vi "Example_OE2031&OE2041 Trig in.vi"() -> ()   [LabVIEW 2011]
panel:
  out "data_buffer":dbl[][](array[numeric])
  out "loss count":i32=-1
  out "cnt":u16
  in  "Ref_Source":u8(ring) items=["External", "Internal"]
  in  "Interval Count":u32=1 min=1 max=100000
  in  "选项卡控件":enum32{"选项卡 "}(tab)
  in  "Sweep Mode":u16(ring) items=["Linear", "Log"]
  in  "Start Frequency(Hz)":dbl=1000.0 min=1e-05 max=60000000.0 format="%#.3f"
  in  "Stop Frequency(Hz)":dbl=5000.0 min=1e-05 max=60000000.0 format="%#.3f"
  in  "Linear Step Frequency(Hz)":dbl=1000.0 min=1e-05 max=60000000.0 format="%#.3f"
  in  "Log Step Percent(%)":dbl=10.0 min=-100.0 max=100.0 format="%#.2f"
  in  "Step Time(ms)":i32=1000 min=50 max=100000
  in  "Sweep Run Mode":u16(ring) items=["Stop", "Singal", "Loop"]
  out "Group":u32
  in  "Sweep":u16(ring) items=["OFF", "ON"]
  in  "function":T1(ring)
  in  "Parameter Index":u16(ring) items=["X", "Y", "R", "θ", "Frequency", "XD1", "YD1", "RD1", "θD1", "XD2", "YD2", "RD2", "θD2", "XD3", "YD3", "RD3", "θD3", "X_Noise", "Y_Noise", "AUXADC1", "AUXADC2", "AUXADC3", "AUXADC4"]
  out "Wave":dbl(graph)
  in  "IP Address":string="192.168.1.10"
  in  "Timeout":u32=100
  in  "Port":u32=10001
  in  "Connect":bool
  in  "Trig Mode":u8(ring) items=["Internal", "Ext_Rissing_Edge", "Ext_Falling_Edge", "Ext_High_Level", "Ext_Low_Level"]
  out "Error out":errorcluster caption="error out"
  in  "Remote Mode":u16(ring) items=["USB"=0, "Ethernet"=3]
  in  "VISA resource name":refnum<visa-resource-name>
  # "Tel          :   +86-020-84133345\nWebsite  :   www.ssi-instrument.com\nE-mail     :   support@si-instrument.com"
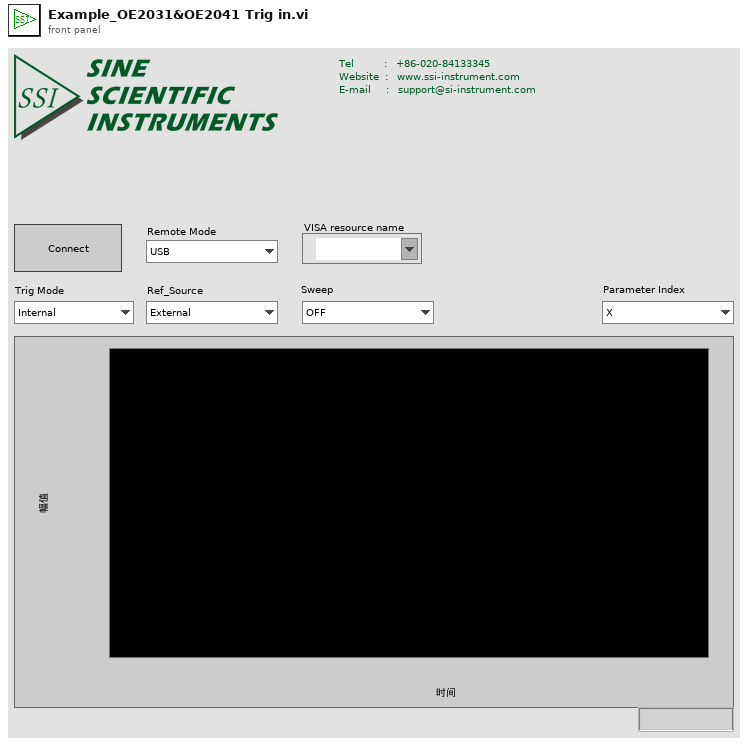
[diagram p1: front panel]
types:
  T1 = enum16{"initial", "Trig In Type", "Sample", "Ext_Sweep_Trig In", "Int_Sweep_Trig In"}
  T2 = enum8{"Enabled", "Disabled", "Disabled and Grayed Out"}
  T3 = cluster{"Port":u32, "Timeout":u32, "IP Address":string}
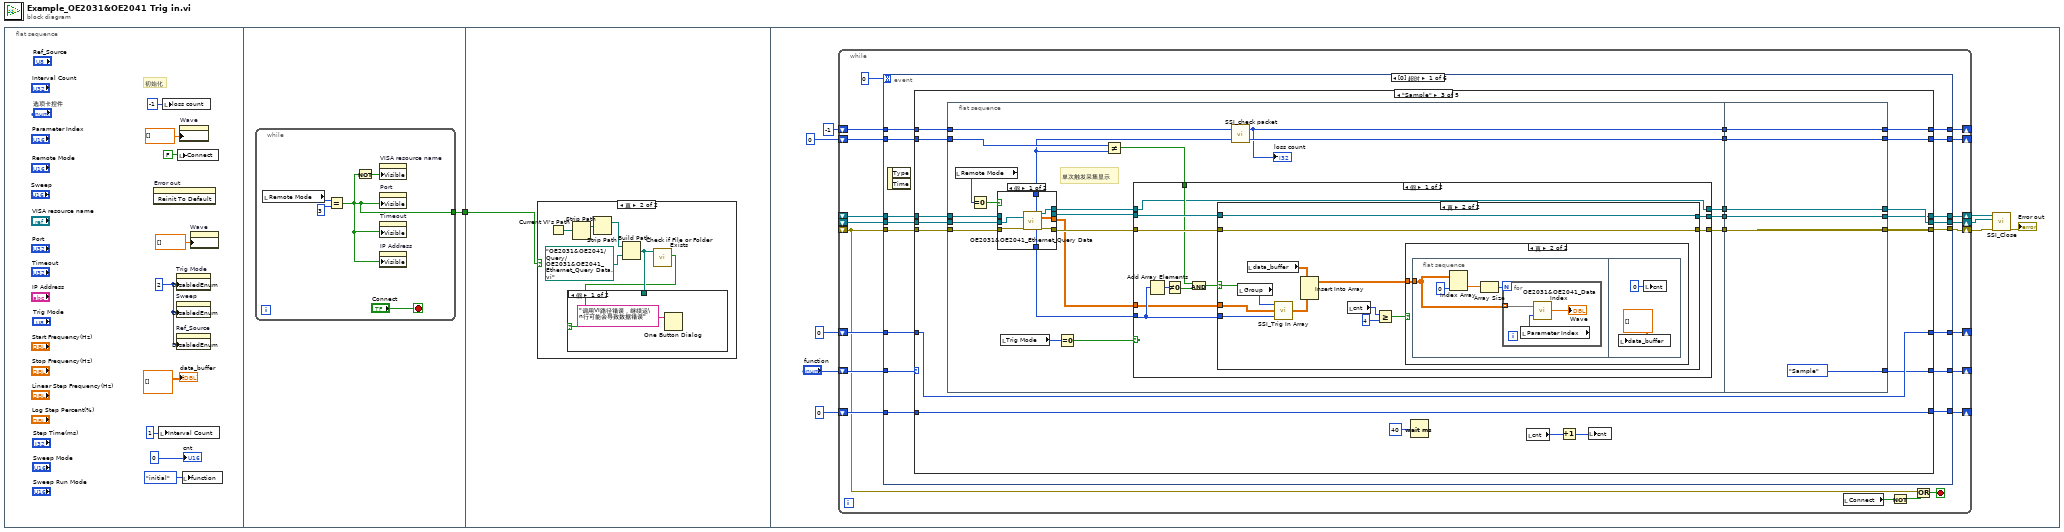
[diagram p0: block diagram]
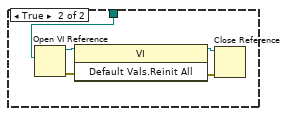
[diagram p3: hidden frame]
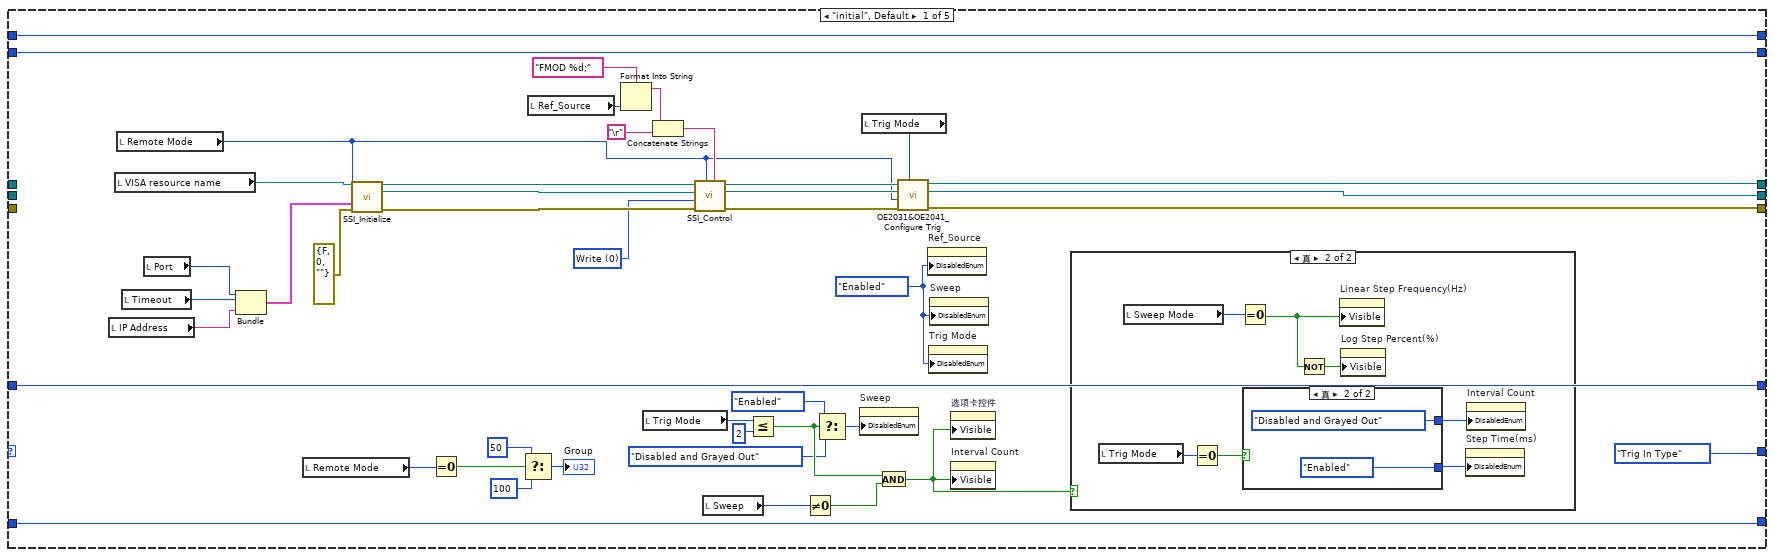
[diagram p4: hidden frame]
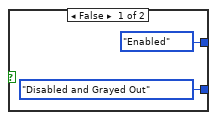
[diagram p6: hidden frame]
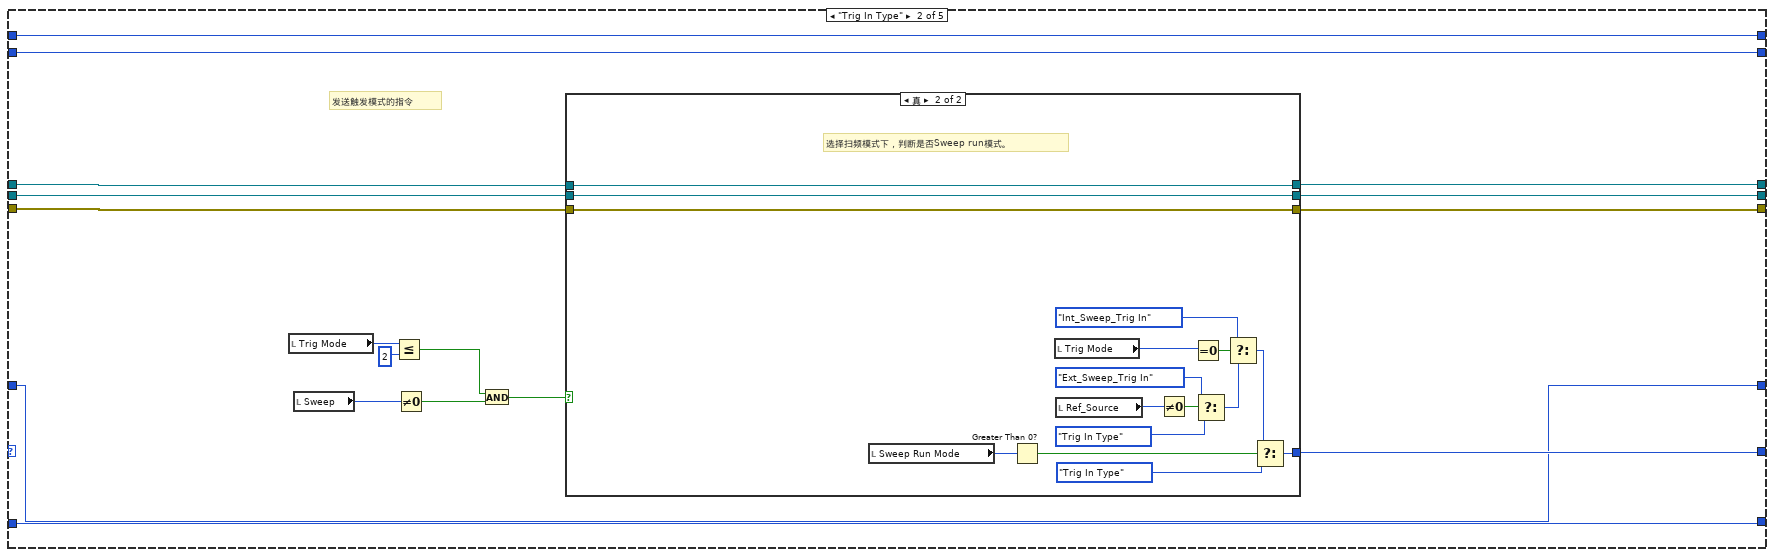
[diagram p7: hidden frame]
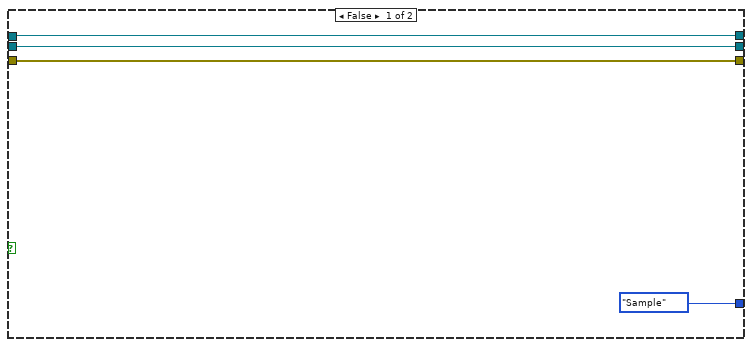
[diagram p8: hidden frame]
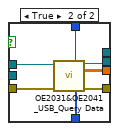
[diagram p9: hidden frame]
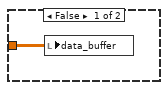
[diagram p11: hidden frame]
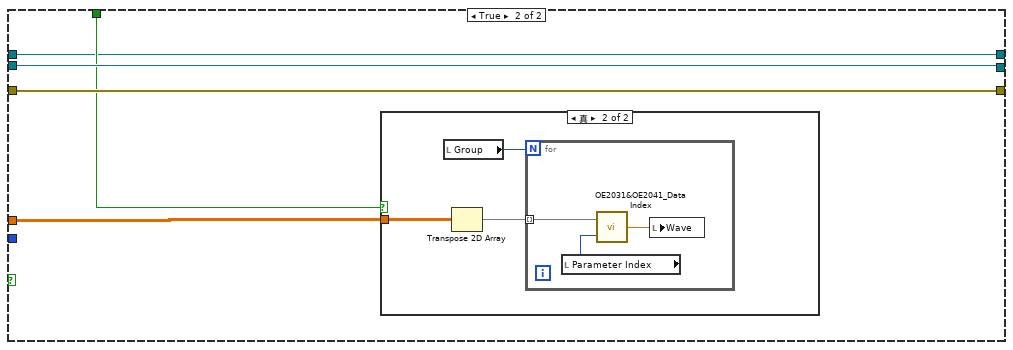
[diagram p12: hidden frame]
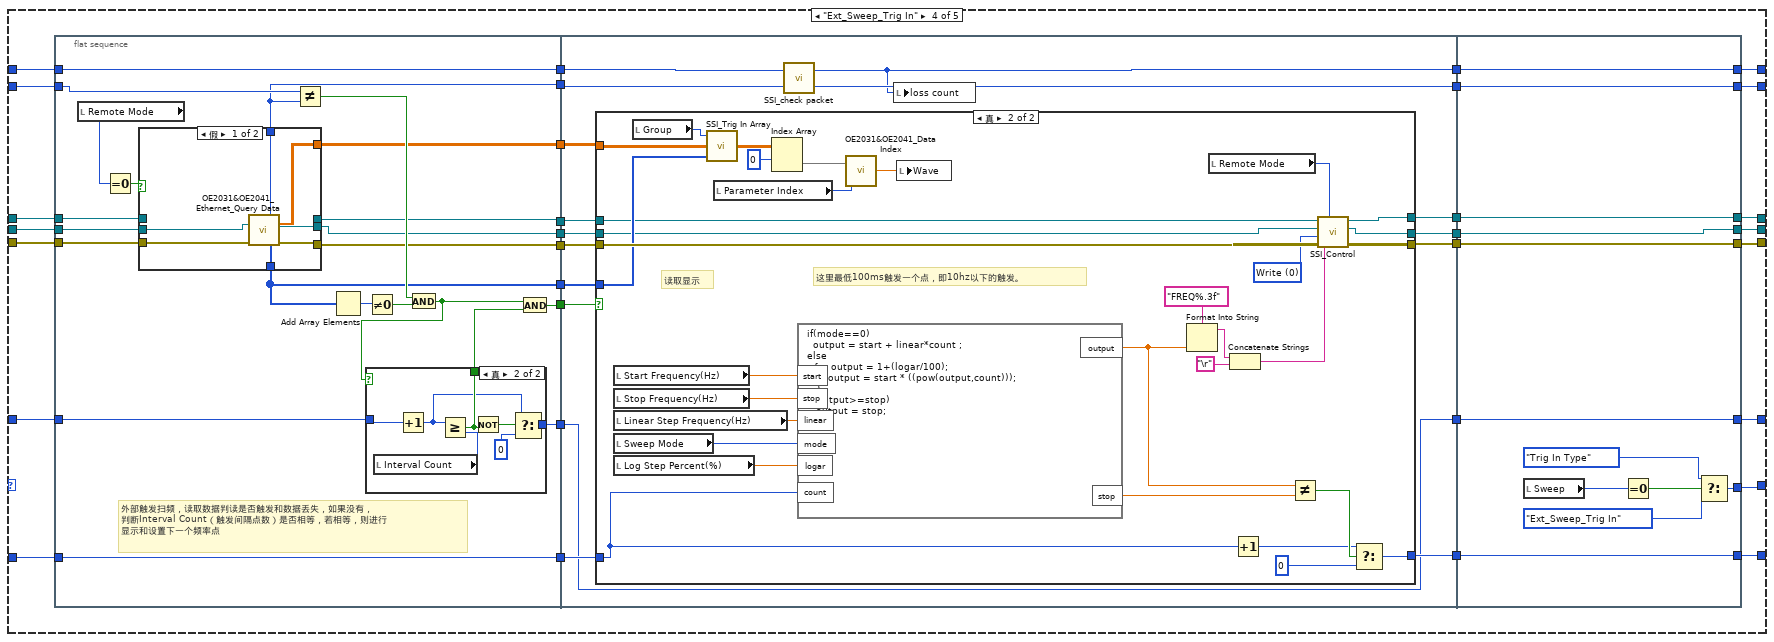
[diagram p14: hidden frame]
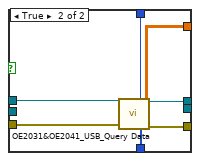
[diagram p15: hidden frame]
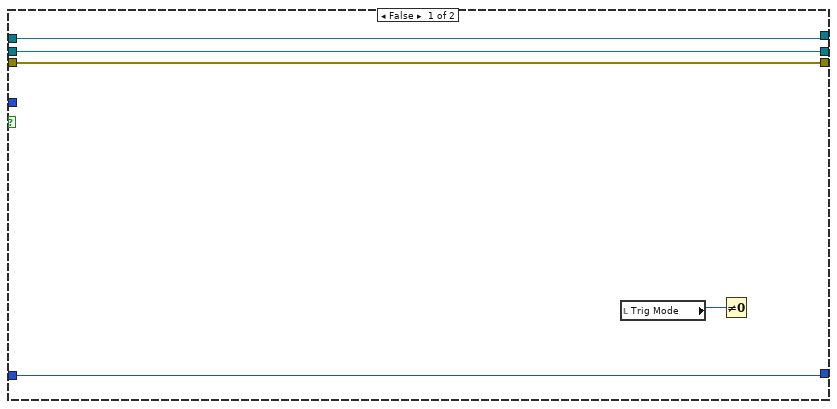
[diagram p17: hidden frame]
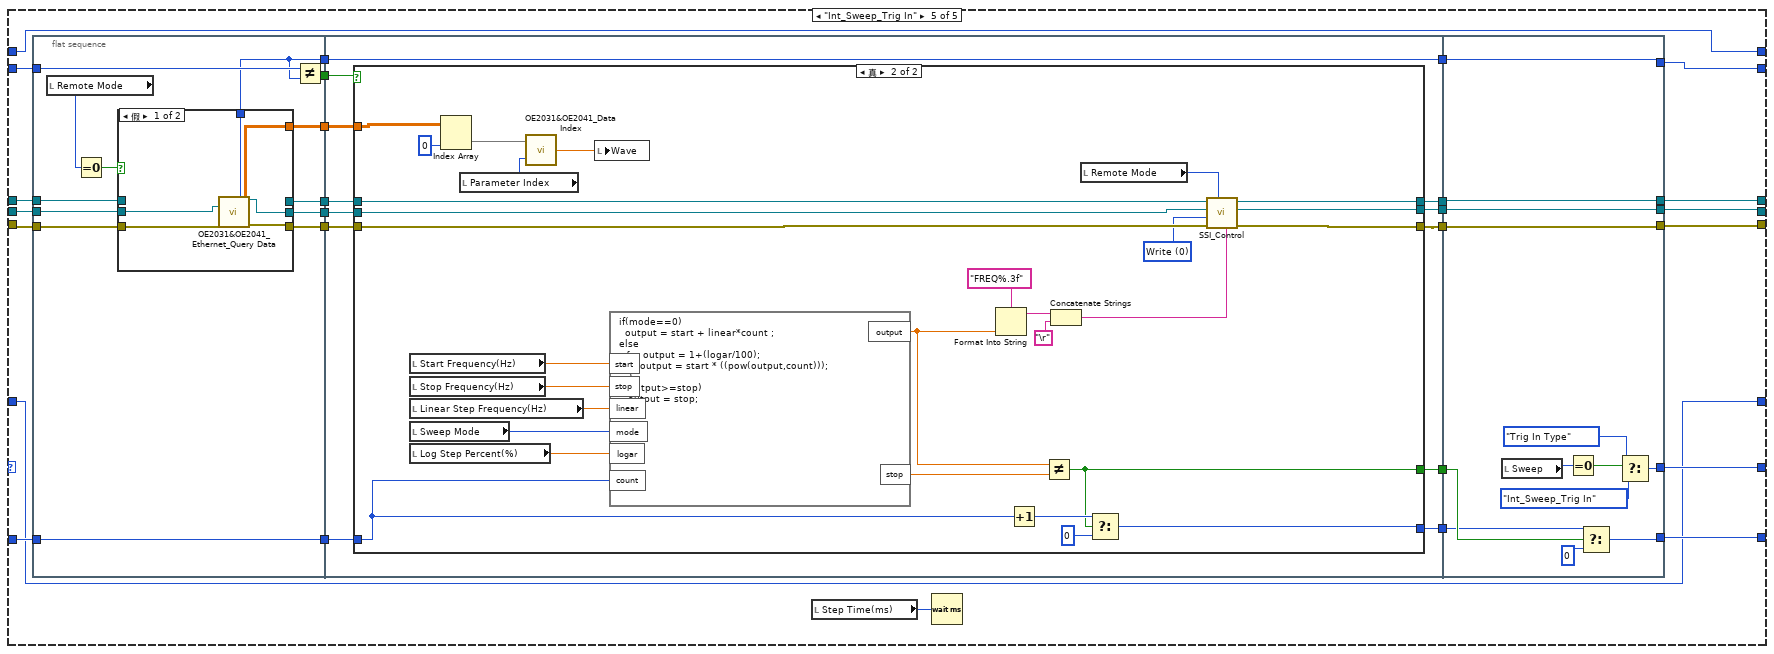
[diagram p18: hidden frame]
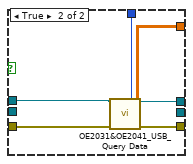
[diagram p19: hidden frame]
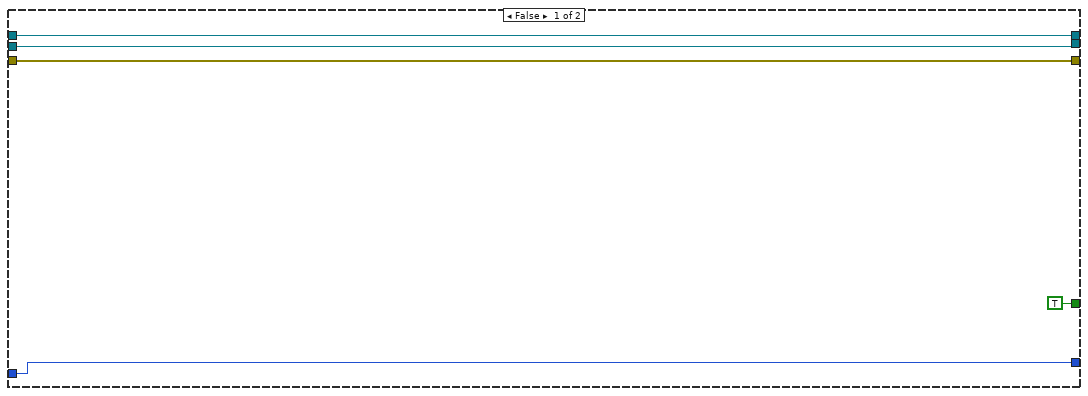
[diagram p20: hidden frame]
diagram:
  n1 = flat-sequence {
    tunnel: [w11] -> w1
    tunnel: w1 -> [w17]
    frame #0 {
      w3 = 2
      # "初始化"
      n2 = invoke on="Error out" class="Clust (严格)" method="Reinit To Default"() -> ()  [unwired: 3 in, 3 out]
      n3 = local write "Interval Count"(u32 1 ("Interval Count")) -> ()
      n4 = local write "loss count"(-1 ("loss count")) -> ()
      n5 = property on="Trig Mode" class="Ring (严格)"("DisabledEnum"=w3) -> ()  [unwired: 2 in, 2 out]
      n6 = property on="Sweep" class="Ring (严格)"("DisabledEnum"=w3) -> ()  [unwired: 2 in, 2 out]
      n7 = property on="Ref_Source" class="Ring (严格)"("DisabledEnum"=w3) -> ()  [unwired: 2 in, 2 out]
      n8 = local write "Connect"(FALSE ("Connect")) -> ()
      n9 = property on="Wave" class="WFChart (严格)"("History Data"=dbl[] [] ("历史数据")) -> ()  [unwired: 2 in, 2 out]
      n10 = local write "function"(T1."initial" ("function")) -> ()
      n11 = property on="Wave" class="WFChart (严格)"("History Data"=dbl[] [] ("历史数据")) -> ()  [unwired: 2 in, 2 out]
      "data_buffer" <- dbl[][] []
      "cnt" <- 0
    }
    frame #1 {
      n12 = while {
        tunnel: [w12] -> w11
        stop <- "Connect" stop-if-true
        n13 = local read "Remote Mode"() -> (w15:u16)
        n14 = Equal?(x=w15, y=u16 3) -> (x = y?=w12:bool)
        n15 = Not(x=w12) -> (.not. x?=w13:bool)
        n16 = property on="VISA resource name" class="VISAName"("Visible"=w13) -> ()  [unwired: 2 in, 2 out]
        n17 = property on="Port" class="DigNum (严格)"("Visible"=w12) -> ()  [unwired: 2 in, 2 out]
        n18 = property on="Timeout" class="DigNum (严格)"("Visible"=w12) -> ()  [unwired: 2 in, 2 out]
        n19 = property on="IP Address" class="Str"("Visible"=w12) -> ()  [unwired: 2 in, 2 out]
      }
    }
    frame #2 {
      n20 = case shown="真" w17 {
        frame False {
        }
        frame True {
          n21 = Current VI's Path() -> (path=w19:path)
          n22 = Strip Path(path=w19) -> (stripped path=w18:path)  [unwired: 1 out]
          n23 = Strip Path(path=w18) -> (stripped path=w20:path)  [unwired: 1 out]
          n24 = Build Path(base path=w20, name or relative path=path "OE2031&OE2041/Query/OE2031&OE2041_Ethernet_Query Data.vi") -> (appended path=w23:path)
          n25 = call <vilib>:"Check if File or Folder Exists.vi"("path"=w23) -> ("file or folder exists?"=w21:bool)  [unwired: 8 in, 2 out]
          n26 = case shown="假" w21 {
            tunnel: w23 -> [_ w29]
            frame False {
              n27 = One Button Dialog(message="调用VI路径错误，继续运\n行可能会导致数据错误" ("消息")) -> ()  [unwired: 1 in, 1 out]
            }
            frame True {
              n28 = Open VI Reference(vi path=w29) -> (vi reference=w26:refnum<vi>, error out=w25:errorcluster)  [unwired: 5 in]
              n29 = invoke class="VI" method="Default Vals.Reinit All"(reference=w26, error in=w25) -> (reference out=w28:refnum<vi>, error out=w27:errorcluster)  [unwired: 1 in, 1 out]
              n30 = Close Reference(reference=w28, error in (no error)=w27) -> ()  [unwired: 1 out]
            }
          }
        }
      }
    }
    frame #3 {
      n31 = while {
        shift-right: [w53] -> _
        shift-left: "function" -> [w54]
        shift-right: [w51] -> _
        shift-left: 0 ("f") -> [w52]
        shift-right: [w48] -> _
        shift-left: 0 -> [w49]
        shift-right: [w45] -> _
        shift-left: 0 -> [w46]
        shift-right: [w42] -> w32
        shift-left: _ -> [w56]
        shift-right: [w55] -> w37
        shift-left: _ -> [w44]
        shift-right: [w43] -> w33
        shift-left: _ -> [w41]
        shift-right: [w39] -> _
        shift-left: -1 ("loss count") -> [w40]
        stop <- w57 stop-if-true
        n32 = event shown="[0] 超时" {
          selector: _ -> [_ _ _ _ _ _]
          dyn-events: _ -> [_ _ _ _ _ _]
          timeout: 0 -> [_ _ _ _ _ _]
          tunnel: w56 -> [w74 w529 w541 w560 w586 w605]
          tunnel: [w73 w529 w541 w555 w585 w605] -> w42
          tunnel: [w72 w527 w540 w557 w588 w606] -> w55
          tunnel: w44 -> [w71 w527 w540 w562 w589 w606]
          tunnel: w54 -> [w70 _ _ _ w592 _]
          tunnel: [w69 T1."Trig In Type" ("function") T1."Trig In Type" ("function") T1."Trig In Type" ("function") w592 T1."Trig In Type" ("function")] -> w53
          tunnel: w52 -> [w68 w533 w543 w567 w593 w601]
          tunnel: [w67 w533 w543 w567 w593 w601] -> w51
          tunnel: w49 -> [w66 w531 w538 w565 w590 w603]
          tunnel: [w65 w531 w538 w565 w590 w603] -> w48
          tunnel: w46 -> [w64 w524 w537 w566 w591 w600]
          tunnel: [w63 w524 w537 w566 w591 w600] -> w45
          tunnel: [w62 w528 w535 w556 w584 w604] -> w43
          tunnel: w41 -> [w61 w528 w535 w561 w587 w604]
          tunnel: w40 -> [w60 w530 w534 w544 w579 w602]
          tunnel: [w59 w530 w534 w544 w579 w602] -> w39
          event Timeout {
            n33 = event-data() -> ()  [unwired: 1 in, 2 out]
            n34 = case shown="\"Sample\"" w70 {
              tunnel: w74 -> [_ w145 w185 w304 w424]
              tunnel: w71 -> [_ w143 w184 w303 w423]
              tunnel: [w96 w144 w168 w300 w437] -> w73
              tunnel: [w94 w142 w176 w301 w436] -> w72
              tunnel: [T1."Trig In Type" ("function") w141 w182 w289 w434] -> w69
              tunnel: w68 -> [w111 w140 w186 w302 w435]
              tunnel: [w111 w140 w186 w299 w433] -> w67
              tunnel: w66 -> [w109 w139 w181 w298 w439]
              tunnel: [w109 w139 w179 w297 w438] -> w65
              tunnel: w64 -> [w110 w138 w183 w284 w432]
              tunnel: [w110 w138 w183 w281 w432] -> w63
              tunnel: [w95 w130 w169 w277 w415] -> w62
              tunnel: w61 -> [_ w131 w171 w280 w419]
              tunnel: w60 -> [w76 w129 w174 w276 w414]
              tunnel: [w76 w129 w167 w273 w414] -> w59
              frame "initial", Default {
                w75 = T2."Enabled" ("禁用")
                w88 = u16 0 items=["Write", "Read"] ("Control")
                n35 = local read "IP Address"() -> (w91:string)
                n36 = local read "VISA resource name"() -> (w97:refnum<visa-resource-name>)
                n37 = local read "Remote Mode"() -> (w77:u16)
                n38 = local read "Timeout"() -> (w92:u32)
                n39 = local read "Port"() -> (w93:u32)
                n40 = Bundle("Port"=w93, "Timeout"=w92, "IP Address"=w91) -> (w90:T3)  [unwired: 1 in]
                n41 = local read "Remote Mode"() -> (w117:u16)
                n42 = call "SSI_Initialize.vi"("VISA resource name"=w97, "Remote Mode"=w77, "Ethernet"=w90, "error in (no error)"=errorcluster {"status"=FALSE, "code"=0, "source"=""}) -> ("VISA resource name out"=w101:refnum<visa-resource-name>, "connection ID(Ethernet)"=w102:refnum<k5>, "error out"=w98:errorcluster)  [unwired: 9 in]
                n43 = Equal To 0?(x=w117) -> (x = 0?=w113:bool)
                n44 = Select(t=50, s=w113, f=100) -> (s? t:f=→"Group":i32)
                n45 = local read "Ref_Source"() -> (w107:u8)
                n46 = Format Into String(format string="FMOD %d;" ("格式字符串"), w107) -> (resulting string=w108:string)  [unwired: 2 in, 1 out]
                n47 = local read "Trig Mode"() -> (w83:u8)
                n48 = Concatenate Strings(w108, "\r") -> (w87:string)
                n49 = call "SSI_Control.vi"("Write Buffer"=w87, "Remote Mode"=w77, "Error in (no error)"=w98, "Control"=w88, "Connection ID in"=w102, "VISA resource name"=w101) -> ("Error out"=w99:errorcluster, "Connection ID out"=w100:refnum<k5>, "VISA resource  out"=w103:refnum<visa-resource-name>)  [unwired: 2 in, 1 out]
                n50 = local read "Sweep"() -> (w84:u16)
                n51 = Less Or Equal?(x=w83, y=u8 2) -> (x <= y?=w85:bool)
                n52 = Not Equal To 0?(x=w84) -> (x != 0?=w86:bool)
                n53 = Select(t=T2."Enabled" ("禁用"), s=w85, f=T2."Disabled and Grayed Out") -> (s? t:f=w80:T2)
                n54 = property on="Sweep" class="Ring (严格)"("DisabledEnum"=w80) -> ()  [unwired: 2 in, 2 out]
                n55 = local read "Trig Mode"() -> (w104:u8)
                n56 = And(x=w85, y=w86) -> (x .and. y?=w78:bool)
                n57 = call "OE2031&OE2041_Configure Trig.vi"("Trig Mode"=w104, "Error in (no error)"=w99, "Remote Mode"=w77, "Connection ID in"=w100, "VISA resource name"=w103) -> ("Error out"=w94:errorcluster, "Connection ID out"=w95:refnum<k5>, "VISA resource  out"=w96:refnum<visa-resource-name>)  [unwired: 3 in, 1 out]
                n58 = property on="Ref_Source" class="Ring (严格)"("DisabledEnum"=w75) -> ()  [unwired: 2 in, 2 out]
                n59 = property on="Trig Mode" class="Ring (严格)"("DisabledEnum"=w75) -> ()  [unwired: 2 in, 2 out]
                n60 = property on="Sweep" class="Ring (严格)"("DisabledEnum"=w75) -> ()  [unwired: 2 in, 2 out]
                n61 = property on="选项卡控件" class="TabCtl (严格)"("Visible"=w78) -> ()  [unwired: 2 in, 2 out]
                n62 = property on="Interval Count" class="DigNum (严格)"("Visible"=w78) -> ()  [unwired: 2 in, 2 out]
                n63 = case shown="真" w78 {
                  frame False {
                  }
                  frame True {
                    n64 = local read "Trig Mode"() -> (w118:u8)
                    n65 = local read "Sweep Mode"() -> (w123:u16)
                    n66 = Equal To 0?(x=w118) -> (x = 0?=w119:bool)
                    n67 = Equal To 0?(x=w123) -> (x = 0?=w124:bool)
                    n68 = case shown="真" w119 {
                      tunnel: [T2."Disabled and Grayed Out" ("禁用") T2."Enabled" ("禁用")] -> w121
                      tunnel: [T2."Enabled" ("禁用") T2."Disabled and Grayed Out" ("禁用")] -> w120
                      frame False {
                      }
                      frame True {
                      }
                    }
                    n69 = Not(x=w124) -> (.not. x?=w122:bool)
                    n70 = property on="Linear Step Frequency(Hz)" class="DigNum (严格)"("Visible"=w124) -> ()  [unwired: 2 in, 2 out]
                    n71 = property on="Log Step Percent(%)" class="DigNum (严格)"("Visible"=w122) -> ()  [unwired: 2 in, 2 out]
                    n72 = property on="Step Time(ms)" class="DigNum (严格)"("DisabledEnum"=w121) -> ()  [unwired: 2 in, 2 out]
                    n73 = property on="Interval Count" class="DigNum (严格)"("DisabledEnum"=w120) -> ()  [unwired: 2 in, 2 out]
                  }
                }
              }
              frame "Trig In Type" {
                # "发送触发模式的指令"
                n74 = local read "Trig Mode"() -> (w135:u8)
                n75 = local read "Sweep"() -> (w134:u16)
                n76 = Less Or Equal?(x=w135, y=u8 2) -> (x <= y?=w133:bool)
                n77 = Not Equal To 0?(x=w134) -> (x != 0?=w132:bool)
                n78 = And(x=w133, y=w132) -> (x .and. y?=w137:bool)
                n79 = case shown="真" w137 {
                  tunnel: [w149 w161] -> w144
                  tunnel: [w148 w160] -> w142
                  tunnel: w143 -> [w148 w160]
                  tunnel: w145 -> [w149 w161]
                  tunnel: [T1."Sample" ("function") w164] -> w141
                  tunnel: w131 -> [w146 w150]
                  tunnel: [w146 w150] -> w130
                  frame False {
                  }
                  frame True {
                    # "选择扫频模式下，判断是否Sweep run模式。"
                    n80 = local read "Sweep Run Mode"() -> (w162:u16)
                    n81 = Greater Than 0?(x=w162) -> (x > 0?=w165:bool)
                    n82 = local read "Trig Mode"() -> (w155:u8)
                    n83 = local read "Ref_Source"() -> (w159:u8)
                    n84 = Not Equal To 0?(x=w159) -> (x != 0?=w158:bool)
                    n85 = Equal To 0?(x=w155) -> (x = 0?=w156:bool)
                    n86 = Select(t=T1."Ext_Sweep_Trig In" ("function"), s=w158, f=T1."Trig In Type" ("function")) -> (s? t:f=w157:T1)
                    n87 = Select(t=T1."Int_Sweep_Trig In" ("function"), s=w156, f=w157) -> (s? t:f=w163:T1)
                    n88 = Select(t=w163, s=w165, f=T1."Trig In Type" ("function")) -> (s? t:f=w164:T1)
                  }
                }
              }
              frame "Sample" {
                n89 = flat-sequence {
                  tunnel: w185 -> [w205]
                  tunnel: w184 -> [w204]
                  tunnel: w181 -> [w201]
                  tunnel: [w197] -> w180
                  tunnel: [w199] -> w178
                  tunnel: [w198] -> w177
                  tunnel: w174 -> [w196]
                  tunnel: w171 -> [w192]
                  tunnel: [w189] -> w170
                  tunnel: [w188] -> w166
                  tunnel: w180 -> [w268]
                  tunnel: w178 -> [w272]
                  tunnel: w177 -> [w271]
                  tunnel: [T1."Sample" ("function")] -> w182
                  tunnel: [w268] -> w179
                  tunnel: [w272] -> w168
                  tunnel: [w271] -> w176
                  tunnel: w170 -> [w269]
                  tunnel: [w269] -> w169
                  tunnel: [w267] -> w167
                  tunnel: w166 -> [w267]
                  frame #0 {
                    # "单次触发采集显示"
                    n90 = local read "Remote Mode"() -> (w193:u16)
                    n91 = Equal To 0?(x=w193) -> (x = 0?=w194:bool)
                    n92 = case shown="假" w194 {
                      tunnel: w205 -> [_ w220]
                      tunnel: w204 -> [w212 w219]
                      tunnel: [w209 w218] -> w202
                      tunnel: [w213 w217] -> w200
                      tunnel: [w208 w216] -> w197
                      tunnel: [w210 w215] -> w195
                      tunnel: w192 -> [w211 _]
                      tunnel: [_ w214] -> w191
                      tunnel: [w207 _] -> w190
                      frame False {
                        n93 = call "OE2031&OE2041_Ethernet_Query Data.vi"("Connection ID in"=w211, "Error in (no error)"=w212) -> ("Buffer Count"=w208:u8, "Connection ID out"=w207:refnum<k5>, "Total Data Array"=w210:dbl[][], "Trig In_Count"=w209:u8[], "Error out"=w213:errorcluster)  [unwired: 6 in, 3 out]
                      }
                      frame True {
                        n94 = call "OE2031&OE2041_USB_Query Data.vi"("VISA resource name"=w220, "Error in (no error)"=w219) -> ("Buffer Count"=w216:u8, "VISA resource  out"=w214:refnum<visa-resource-name>, "Total Data Array"=w215:dbl[][], "Trig In_Count"=w218:u8[], "Error out"=w217:errorcluster)  [unwired: 6 in, 3 out]
                      }
                    }
                    n95 = local read "Trig Mode"() -> (w206:u8)
                    n96 = Equal To 0?(x=w206) -> (x = 0?=w203:bool)
                    n97 = Not Equal?(x=w201, y=w197) -> (x != y?=w187:bool)
                    n98 = case shown="假" w203 {
                      tunnel: w195 -> [w223 w258]
                      tunnel: w202 -> [w230 _]
                      tunnel: w187 -> [w222 w257]
                      tunnel: w200 -> [w225 w259]
                      tunnel: w191 -> [w227 w260]
                      tunnel: [w226 w260] -> w199
                      tunnel: [w224 w259] -> w198
                      tunnel: w190 -> [w221 w256]
                      tunnel: [w221 w256] -> w189
                      frame False {
                        n99 = Add Array Elements(numeric array=w230) -> (sum=w231:u8)
                        n100 = Not Equal To 0?(x=w231) -> (x != 0?=w229:bool)
                        n101 = And(x=w222, y=w229) -> (x .and. y?=w228:bool)
                        n102 = case shown="真" w228 {
                          tunnel: w223 -> [_ w242]
                          tunnel: w230 -> [_ w241]
                          tunnel: [w233 w244] -> w226
                          tunnel: w227 -> [w233 w244]
                          tunnel: w225 -> [w232 w243]
                          tunnel: [w232 w243] -> w224
                          frame False {
                          }
                          frame True {
                            n103 = local read "Group"() -> (w240:u32)
                            n104 = local read "data_buffer"() -> (w239:dbl[][])
                            n105 = call "SSI_Trig In Array.vi"("Trig_Count"=w241, "Input Array"=w242, "Group"=w240) -> ("Output Array"=w238:dbl[][])
                            n106 = Insert Into Array(array=w239, new element=w238) -> (w237:dbl[][])  [unwired: 2 in]
                            n107 = local read "cnt"() -> (w236:u16)
                            n108 = Greater Or Equal?(x=w236, y=u16 4) -> (x >= y?=w234:bool)
                            n109 = case shown="真" w234 {
                              tunnel: w237 -> [w245 w246]
                              frame False {
                                n110 = local write "data_buffer"(w245) -> ()
                              }
                              frame True {
                                n111 = flat-sequence {
                                tunnel: w246 -> [w248]
                                frame #0 {
                                n112 = Index Array(array=w248, index (col)=0 ("禁用的索引 (列)")) -> (element=w247:dbl[])  [unwired: 1 in]
                                n113 = Array Size(array=w247) -> (size(s)=w250:i32)
                                n114 = for {
                                N: w250 -> [_]
                                tunnel: w248 -> [w251] mode=indexing
                                n115 = local read "Parameter Index"() -> (w253:u16)
                                n116 = call "OE2031&OE2041_Data Index.vi"("Parameter Type"=w253, "Input Date Array"=w251) -> ("Parameter"=→"Wave":dbl)
                                }
                                }
                                frame #1 {
                                n117 = local write "data_buffer"(dbl[][] [] ("data_buffer")) -> ()
                                n118 = local write "cnt"(u16 0 ("cnt")) -> ()
                                }
                                }
                              }
                            }
                          }
                        }
                      }
                      frame True {
                        n119 = case shown="真" w257 {
                          tunnel: w258 -> [_ w263]
                          frame False {
                          }
                          frame True {
                            n120 = local read "Group"() -> (w262:u32)
                            n121 = Transpose 2D Array(2D array=w263) -> (transposed array=w261:dbl[][])
                            n122 = for {
                              N: w262 -> [_]
                              tunnel: w261 -> [w265] mode=indexing
                              n123 = local read "Parameter Index"() -> (w266:u16)
                              n124 = call "OE2031&OE2041_Data Index.vi"("Parameter Type"=w266, "Input Date Array"=w265) -> ("Parameter"=w264:dbl)
                              n125 = local write "Wave"(w264) -> ()
                            }
                          }
                        }
                      }
                    }
                    n126 = call "SSI_check packet.vi"("input"=w197, "input loss"=w196) -> ("loss count"=w188:i32)  [unwired: 1 out]
                    "loss count" <- w188
                  }
                  frame #1 {
                  }
                }
                n127 = Wait (ms)(milliseconds to wait=40) -> ()  [unwired: 1 out]
                n128 = local read "cnt"() -> (w172:u16)
                n129 = Increment(x=w172) -> (x+1=w173:u16)
                n130 = local write "cnt"(w173) -> ()
              }
              frame "Ext_Sweep_Trig In" {
                n131 = flat-sequence {
                  tunnel: w304 -> [w325]
                  tunnel: w303 -> [w324]
                  tunnel: w302 -> [w322]
                  tunnel: [w318] -> w296
                  tunnel: w298 -> [w326]
                  tunnel: [w322] -> w295
                  tunnel: [w323] -> w294
                  tunnel: [w317] -> w288
                  tunnel: [w316] -> w287
                  tunnel: [w315] -> w286
                  tunnel: [w314] -> w285
                  tunnel: w284 -> [w312]
                  tunnel: [w310] -> w283
                  tunnel: w280 -> [w307]
                  tunnel: [w306] -> w279
                  tunnel: w276 -> [w305]
                  tunnel: [w305] -> w275
                  tunnel: w296 -> [w363]
                  tunnel: w294 -> [w350]
                  tunnel: w295 -> [w359]
                  tunnel: [w360] -> w293
                  tunnel: [w361] -> w292
                  tunnel: [w358] -> w291
                  tunnel: [w350] -> w290
                  tunnel: w288 -> [w362]
                  tunnel: w287 -> [w357]
                  tunnel: w286 -> [w356]
                  tunnel: w285 -> [w355]
                  tunnel: w283 -> [w354]
                  tunnel: [w354] -> w282
                  tunnel: w279 -> [w353]
                  tunnel: [w352] -> w278
                  tunnel: w275 -> [w351]
                  tunnel: [w349] -> w274
                  tunnel: [w411] -> w297
                  tunnel: [w412] -> w299
                  tunnel: [w409] -> w300
                  tunnel: [w410] -> w301
                  tunnel: w293 -> [w410]
                  tunnel: w292 -> [w409]
                  tunnel: w291 -> [w412]
                  tunnel: w290 -> [w411]
                  tunnel: [w407] -> w289
                  tunnel: w282 -> [w408]
                  tunnel: [w408] -> w281
                  tunnel: w278 -> [w402]
                  tunnel: [w402] -> w277
                  tunnel: w274 -> [w401]
                  tunnel: [w401] -> w273
                  frame #0 {
                    # "外部触发扫频，读取数据判读是否触发和数据丢失，如果没有，\n判断Interval Count（触发间隔点数）是否相等，若相等，则进行\n显示和设置下一个频率点"
                    n132 = local read "Remote Mode"() -> (w308:u16)
                    n133 = Equal To 0?(x=w308) -> (x = 0?=w309:bool)
                    n134 = case shown="假" w309 {
                      tunnel: w325 -> [_ w340]
                      tunnel: w324 -> [w333 w339]
                      tunnel: [w329 w338] -> w323
                      tunnel: [_ w337] -> w318
                      tunnel: [w332 w336] -> w317
                      tunnel: [w330 w335] -> w316
                      tunnel: [w328 w334] -> w315
                      tunnel: [w331 _] -> w306
                      tunnel: w307 -> [w327 _]
                      frame False {
                        n135 = call "OE2031&OE2041_Ethernet_Query Data.vi"("Connection ID in"=w327, "Error in (no error)"=w333) -> ("Buffer Count"=w329:u8, "Connection ID out"=w331:refnum<k5>, "Total Data Array"=w330:dbl[][], "Trig In_Count"=w328:u8[], "Error out"=w332:errorcluster)  [unwired: 6 in, 3 out]
                      }
                      frame True {
                        n136 = call "OE2031&OE2041_USB_Query Data.vi"("VISA resource name"=w340, "Error in (no error)"=w339) -> ("Buffer Count"=w338:u8, "VISA resource  out"=w337:refnum<visa-resource-name>, "Total Data Array"=w335:dbl[][], "Trig In_Count"=w334:u8[], "Error out"=w336:errorcluster)  [unwired: 6 in, 3 out]
                      }
                    }
                    n137 = Not Equal?(x=w326, y=w323) -> (x != y?=w320:bool)
                    n138 = Add Array Elements(numeric array=w315) -> (sum=w321:u8)
                    n139 = Not Equal To 0?(x=w321) -> (x != 0?=w319:bool)
                    n140 = And(x=w320, y=w319) -> (x .and. y?=w313:bool)
                    n141 = case shown="真" w313 {
                      tunnel: w312 -> [w341 w348]
                      tunnel: [_ w345] -> w311
                      tunnel: [w341 w342] -> w310
                      frame False {
                      }
                      frame True {
                        n142 = local read "Interval Count"() -> (w347:u32)
                        n143 = Increment(x=w348) -> (x+1=w344:i32)
                        n144 = Greater Or Equal?(x=w344, y=w347) -> (x >= y?=w345:bool)
                        n145 = Not(x=w345) -> (.not. x?=w346:bool)
                        n146 = Select(t=w344, s=w346, f=0) -> (s? t:f=w342:i32)
                      }
                    }
                    n147 = And(x=w313, y=w311) -> (x .and. y?=w314:bool)
                  }
                  frame #1 {
                    n148 = case shown="真" w355 {
                      tunnel: w362 -> [w367 w383]
                      tunnel: [w367 w385] -> w360
                      tunnel: [w368 w370] -> w361
                      tunnel: w363 -> [w368 w371]
                      tunnel: w359 -> [w366 w391]
                      tunnel: [w366 w390] -> w358
                      tunnel: w357 -> [_ w381]
                      tunnel: w356 -> [_ w379]
                      tunnel: w353 -> [w364 w375]
                      tunnel: [w364 w374] -> w352
                      frame False {
                        n149 = local read "Trig Mode"() -> (w365:u8)
                        n150 = Not Equal To 0?(x=w365) -> ()  [unwired: 1 out]
                      }
                      frame True {
                        w372 = u16 0 items=["Write", "Read"] ("Control")
                        # "这里最低100ms触发一个点，即10hz以下的触发。"
                        # "读取显示"
                        n151 = local read "Start Frequency(Hz)"() -> (w397:dbl)
                        n152 = local read "Stop Frequency(Hz)"() -> (w396:dbl)
                        n153 = local read "Linear Step Frequency(Hz)"() -> (w395:dbl)
                        n154 = local read "Sweep Mode"() -> (w394:u16)
                        n155 = local read "Log Step Percent(%)"() -> (w393:dbl)
                        n156 = local read "Group"() -> (w380:u32)
                        n157 = call "SSI_Trig In Array.vi"("Trig_Count"=w379, "Input Array"=w381, "Group"=w380) -> ("Output Array"=w378:dbl[][])
                        n158 = local read "Parameter Index"() -> (w382:u16)
                        n159 = Index Array(array=w378, index (row)=0 ("索引 (行)")) -> (element=w376:dbl[])  [unwired: 1 in]
                        n160 = formula code="if(mode==0)\n  output = start + linear*count ;\nelse \n  {    output = 1+(logar/100);\n       output = start * ((pow(output,count)));\n   }\nif(output>=stop)\n   output = stop;"("start"=w397, "stop"=w396, "linear"=w395, "logar"=w393, "mode"=w394, "count"=w391) -> ("stop"=w392:dbl, "output"=w386:dbl)
                        n161 = call "OE2031&OE2041_Data Index.vi"("Parameter Type"=w382, "Input Date Array"=w376) -> ("Parameter"=w377:dbl)
                        n162 = local write "Wave"(w377) -> ()
                        n163 = Format Into String(format string="FREQ%.3f" ("格式字符串"), w386) -> (resulting string=w399:string)  [unwired: 2 in, 1 out]
                        n164 = local read "Remote Mode"() -> (w373:u16)
                        n165 = Concatenate Strings(w399, "\r") -> (w384:string)
                        n166 = Increment(x=w391) -> (x+1=w388:i32)
                        n167 = Not Equal?(x=w386, y=w392) -> (x != y?=w389:bool)
                        n168 = call "SSI_Control.vi"("Write Buffer"=w384, "Remote Mode"=w373, "Error in (no error)"=w383, "Control"=w372, "Connection ID in"=w375, "VISA resource name"=w371) -> ("Error out"=w385:errorcluster, "Connection ID out"=w374:refnum<k5>, "VISA resource  out"=w370:refnum<visa-resource-name>)  [unwired: 2 in, 1 out]
                        n169 = Select(t=w388, s=w389, f=0) -> (s? t:f=w390:i32)
                      }
                    }
                    n170 = call "SSI_check packet.vi"("input"=w350, "input loss"=w351) -> ("loss count"=w349:i32)  [unwired: 1 out]
                    n171 = local write "loss count"(w349) -> ()
                  }
                  frame #2 {
                    n172 = local read "Sweep"() -> (w406:u16)
                    n173 = Equal To 0?(x=w406) -> (x = 0?=w405:bool)
                    n174 = Select(t=T1."Trig In Type" ("function"), s=w405, f=T1."Ext_Sweep_Trig In" ("function")) -> (s? t:f=w407:T1)
                  }
                }
              }
              frame "Int_Sweep_Trig In" {
                n175 = flat-sequence {
                  tunnel: [w449] -> w431
                  tunnel: [w444] -> w429
                  tunnel: [w448] -> w427
                  tunnel: w439 -> [w452]
                  tunnel: w435 -> [w450]
                  tunnel: w424 -> [w445]
                  tunnel: w423 -> [w447]
                  tunnel: [w451] -> w422
                  tunnel: [w450] -> w421
                  tunnel: w419 -> [w446]
                  tunnel: [w443] -> w418
                  tunnel: [w440] -> w417
                  tunnel: w431 -> [w476]
                  tunnel: [w476] -> w430
                  tunnel: w429 -> [w475]
                  tunnel: [w474] -> w428
                  tunnel: w427 -> [w473]
                  tunnel: [w472] -> w426
                  tunnel: [w468] -> w425
                  tunnel: w422 -> [w471]
                  tunnel: w421 -> [w470]
                  tunnel: [w469] -> w420
                  tunnel: w418 -> [w467]
                  tunnel: w417 -> [w466]
                  tunnel: [w465] -> w416
                  tunnel: [w523] -> w438
                  tunnel: w430 -> [w523]
                  tunnel: w428 -> [w522]
                  tunnel: [w522] -> w437
                  tunnel: [w521] -> w436
                  tunnel: w426 -> [w521]
                  tunnel: [w514] -> w434
                  tunnel: [w520] -> w433
                  tunnel: w425 -> [w518]
                  tunnel: w420 -> [w517]
                  tunnel: w416 -> [w511]
                  tunnel: [w511] -> w415
                  frame #0 {
                    n176 = local read "Remote Mode"() -> (w441:u16)
                    n177 = Equal To 0?(x=w441) -> (x = 0?=w442:bool)
                    n178 = case shown="假" w442 {
                      tunnel: [w456 w464] -> w449
                      tunnel: [_ w463] -> w444
                      tunnel: [w458 w462] -> w448
                      tunnel: [w457 w461] -> w443
                      tunnel: w447 -> [w455 w459]
                      tunnel: w446 -> [w454 _]
                      tunnel: w445 -> [_ w460]
                      tunnel: [w453 _] -> w440
                      frame False {
                        n179 = call "OE2031&OE2041_Ethernet_Query Data.vi"("Connection ID in"=w454, "Error in (no error)"=w455) -> ("Buffer Count"=w456:u8, "Connection ID out"=w453:refnum<k5>, "Total Data Array"=w457:dbl[][], "Error out"=w458:errorcluster)  [unwired: 6 in, 4 out]
                      }
                      frame True {
                        n180 = call "OE2031&OE2041_USB_Query Data.vi"("VISA resource name"=w460, "Error in (no error)"=w459) -> ("Buffer Count"=w464:u8, "VISA resource  out"=w463:refnum<visa-resource-name>, "Total Data Array"=w461:dbl[][], "Error out"=w462:errorcluster)  [unwired: 6 in, 4 out]
                      }
                    }
                    n181 = Not Equal?(x=w452, y=w449) -> (x != y?=w451:bool)
                  }
                  frame #1 {
                    n182 = case shown="真" w471 {
                      tunnel: w475 -> [w481 w484]
                      tunnel: [w481 w483] -> w474
                      tunnel: [w480 w490] -> w472
                      tunnel: w473 -> [w480 w491]
                      tunnel: w470 -> [w479 w504]
                      tunnel: [w479 w498] -> w469
                      tunnel: [TRUE w499] -> w468
                      tunnel: w467 -> [_ w487]
                      tunnel: w466 -> [w477 w486]
                      tunnel: [w477 w482] -> w465
                      frame False {
                      }
                      frame True {
                        w485 = u16 0 items=["Write", "Read"] ("Control")
                        n183 = local read "Start Frequency(Hz)"() -> (w510:dbl)
                        n184 = local read "Stop Frequency(Hz)"() -> (w509:dbl)
                        n185 = local read "Linear Step Frequency(Hz)"() -> (w508:dbl)
                        n186 = local read "Sweep Mode"() -> (w507:u16)
                        n187 = local read "Log Step Percent(%)"() -> (w506:dbl)
                        n188 = Index Array(array=w487, index (col)=0 ("禁用的索引 (列)")) -> (element=w492:dbl[])  [unwired: 1 in]
                        n189 = local read "Parameter Index"() -> (w495:u16)
                        n190 = call "OE2031&OE2041_Data Index.vi"("Parameter Type"=w495, "Input Date Array"=w492) -> ("Parameter"=w494:dbl)
                        n191 = local write "Wave"(w494) -> ()
                        n192 = formula code="if(mode==0)\n  output = start + linear*count ;\nelse \n  {    output = 1+(logar/100);\n       output = start * ((pow(output,count)));\n   }\nif(output>=stop)\n   output = stop;"("start"=w510, "stop"=w509, "linear"=w508, "logar"=w506, "mode"=w507, "count"=w504) -> ("stop"=w500:dbl, "output"=w496:dbl)
                        n193 = Format Into String(format string="FREQ%.3f" ("格式字符串"), w496) -> (resulting string=w501:string)  [unwired: 2 in, 1 out]
                        n194 = Increment(x=w504) -> (x+1=w505:i32)
                        n195 = Not Equal?(x=w496, y=w500) -> (x != y?=w499:bool)
                        n196 = Concatenate Strings(w501, "\r") -> (w489:string)
                        n197 = local read "Remote Mode"() -> (w488:u16)
                        n198 = Select(t=w505, s=w499, f=0) -> (s? t:f=w498:i32)
                        n199 = call "SSI_Control.vi"("Write Buffer"=w489, "Remote Mode"=w488, "Error in (no error)"=w491, "Control"=w485, "Connection ID in"=w486, "VISA resource name"=w484) -> ("Error out"=w490:errorcluster, "Connection ID out"=w482:refnum<k5>, "VISA resource  out"=w483:refnum<visa-resource-name>)  [unwired: 2 in, 1 out]
                      }
                    }
                  }
                  frame #2 {
                    n200 = local read "Sweep"() -> (w516:u16)
                    n201 = Equal To 0?(x=w516) -> (x = 0?=w515:bool)
                    n202 = Select(t=w517, s=w518, f=u16 0) -> (s? t:f=w520:i32)
                    n203 = Select(t=T1."Trig In Type" ("function"), s=w515, f=T1."Int_Sweep_Trig In" ("function")) -> (s? t:f=w514:T1)
                  }
                }
                n204 = local read "Step Time(ms)"() -> (w413:i32)
                n205 = Wait (ms)(milliseconds to wait=w413) -> ()  [unwired: 1 out]
              }
            }
          }
          event "Stop Frequency(Hz)", "Linear Step Frequency(Hz)", "Log Step Percent(%)", "Sweep Run Mode", "Sweep Mode", "Start Frequency(Hz)": Value Change {
            n206 = event-data() -> ()  [unwired: 1 in, 5 out]
            n207 = property on="Wave" class="WFChart (严格)"("History Data"=dbl[] [] ("历史数据")) -> ()  [unwired: 2 in, 2 out]
            n208 = Wait (ms)(milliseconds to wait=u32 10 ("等待时间（毫秒）")) -> ()  [unwired: 1 out]
          }
          event "Parameter Index": Value Change {
            n209 = event-data() -> ()  [unwired: 1 in, 5 out]
            n210 = property on="Wave" class="WFChart (严格)"("History Data"=dbl[] [] ("历史数据")) -> ()  [unwired: 2 in, 2 out]
            n211 = Wait (ms)(milliseconds to wait=u32 10 ("等待时间（毫秒）")) -> ()  [unwired: 1 out]
          }
          event "Trig Mode": Value Change {
            n212 = event-data() -> ()  [unwired: 1 in, 5 out]
            n213 = local read "Trig Mode"() -> (w558:u8)
            n214 = local read "Remote Mode"() -> (w559:u16)
            n215 = call "OE2031&OE2041_Configure Trig.vi"("Trig Mode"=w558, "Error in (no error)"=w562, "Remote Mode"=w559, "Connection ID in"=w561, "VISA resource name"=w560) -> ("Error out"=w557:errorcluster, "Connection ID out"=w556:refnum<k5>, "VISA resource  out"=w555:refnum<visa-resource-name>)  [unwired: 3 in, 1 out]
            n216 = local read "Trig Mode"() -> (w550:u8)
            n217 = local read "Sweep"() -> (w546:u16)
            n218 = Less Or Equal?(x=w550, y=u8 2) -> (x <= y?=w549:bool)
            n219 = Select(t=T2."Enabled" ("禁用"), s=w549, f=T2."Disabled and Grayed Out") -> (s? t:f=w553:T2)
            n220 = property on="Wave" class="WFChart (严格)"("History Data"=dbl[] [] ("历史数据")) -> ()  [unwired: 2 in, 2 out]
            n221 = Not Equal To 0?(x=w546) -> (x != 0?=w545:bool)
            n222 = property on="Sweep" class="Ring (严格)"("DisabledEnum"=w553) -> ()  [unwired: 2 in, 2 out]
            n223 = And(x=w549, y=w545) -> (x .and. y?=w548:bool)
            n224 = Wait (ms)(milliseconds to wait=u32 10 ("等待时间（毫秒）")) -> ()  [unwired: 1 out]
            n225 = property on="选项卡控件" class="TabCtl (严格)"("Visible"=w548) -> ()  [unwired: 2 in, 2 out]
            n226 = property on="Interval Count" class="DigNum (严格)"("Visible"=w548) -> ()  [unwired: 2 in, 2 out]
            n227 = case shown="真" w548 {
              frame False {
              }
              frame True {
                n228 = local read "Trig Mode"() -> (w568:u8)
                n229 = local read "Sweep Mode"() -> (w573:u16)
                n230 = Equal To 0?(x=w568) -> (x = 0?=w569:bool)
                n231 = Equal To 0?(x=w573) -> (x = 0?=w574:bool)
                n232 = case shown="真" w569 {
                  tunnel: [T2."Disabled and Grayed Out" ("禁用") T2."Enabled" ("禁用")] -> w571
                  tunnel: [T2."Enabled" ("禁用") T2."Disabled and Grayed Out" ("禁用")] -> w570
                  frame False {
                  }
                  frame True {
                  }
                }
                n233 = Not(x=w574) -> (.not. x?=w572:bool)
                n234 = property on="Linear Step Frequency(Hz)" class="DigNum (严格)"("Visible"=w574) -> ()  [unwired: 2 in, 2 out]
                n235 = property on="Log Step Percent(%)" class="DigNum (严格)"("Visible"=w572) -> ()  [unwired: 2 in, 2 out]
                n236 = property on="Step Time(ms)" class="DigNum (严格)"("DisabledEnum"=w571) -> ()  [unwired: 2 in, 2 out]
                n237 = property on="Interval Count" class="DigNum (严格)"("DisabledEnum"=w570) -> ()  [unwired: 2 in, 2 out]
              }
            }
          }
          event "Ref_Source": Value Change {
            w597 = u16 0 items=["Write", "Read"] ("Control")
            n238 = event-data() -> ()  [unwired: 1 in, 5 out]
            n239 = local read "Remote Mode"() -> (w583:u16)
            n240 = local read "Ref_Source"() -> (w595:u8)
            n241 = Format Into String(format string="FMOD %d;" ("格式字符串"), w595) -> (resulting string=w594:string)  [unwired: 2 in, 1 out]
            n242 = Concatenate Strings(w594, "\r") -> (w598:string)
            n243 = property on="Wave" class="WFChart (严格)"("History Data"=dbl[] [] ("历史数据")) -> ()  [unwired: 2 in, 2 out]
            n244 = call "SSI_Control.vi"("Write Buffer"=w598, "Remote Mode"=w583, "Error in (no error)"=w589, "Control"=w597, "Connection ID in"=w587, "VISA resource name"=w586) -> ("Error out"=w588:errorcluster, "Connection ID out"=w584:refnum<k5>, "VISA resource  out"=w585:refnum<visa-resource-name>)  [unwired: 2 in, 1 out]
            n245 = Wait (ms)(milliseconds to wait=u32 10 ("等待时间（毫秒）")) -> ()  [unwired: 1 out]
          }
          event "Sweep": Value Change {
            n246 = event-data() -> ()  [unwired: 1 in, 5 out]
            n247 = local read "Sweep"() -> (w608:u16)
            n248 = Not Equal To 0?(x=w608) -> (x != 0?=w599:bool)
            n249 = case shown="真" w599 {
              frame False {
              }
              frame True {
                n250 = local read "Trig Mode"() -> (w610:u8)
                n251 = local read "Sweep Mode"() -> (w615:u16)
                n252 = Equal To 0?(x=w610) -> (x = 0?=w611:bool)
                n253 = Equal To 0?(x=w615) -> (x = 0?=w616:bool)
                n254 = case shown="真" w611 {
                  tunnel: [T2."Disabled and Grayed Out" ("禁用") T2."Enabled" ("禁用")] -> w613
                  tunnel: [T2."Enabled" ("禁用") T2."Disabled and Grayed Out" ("禁用")] -> w612
                  frame False {
                  }
                  frame True {
                  }
                }
                n255 = Not(x=w616) -> (.not. x?=w614:bool)
                n256 = property on="Linear Step Frequency(Hz)" class="DigNum (严格)"("Visible"=w616) -> ()  [unwired: 2 in, 2 out]
                n257 = property on="Log Step Percent(%)" class="DigNum (严格)"("Visible"=w614) -> ()  [unwired: 2 in, 2 out]
                n258 = property on="Step Time(ms)" class="DigNum (严格)"("DisabledEnum"=w613) -> ()  [unwired: 2 in, 2 out]
                n259 = property on="Interval Count" class="DigNum (严格)"("DisabledEnum"=w612) -> ()  [unwired: 2 in, 2 out]
              }
            }
            n260 = property on="选项卡控件" class="TabCtl (严格)"("Visible"=w599) -> ()  [unwired: 2 in, 2 out]
            n261 = property on="Interval Count" class="DigNum (严格)"("Visible"=w599) -> ()  [unwired: 2 in, 2 out]
            n262 = property on="Wave" class="WFChart (严格)"("History Data"=dbl[] [] ("历史数据")) -> ()  [unwired: 2 in, 2 out]
          }
        }
        n263 = local read "Connect"() -> (w47:bool)
        n264 = Not(x=w47) -> (.not. x?=w58:bool)
        n265 = Or(x=w44, y=w58) -> (x .or. y?=w57:bool)
      }
      n266 = call "SSI_Close.vi"("Error in (no error)"=w37, "Connection ID in"=w33, "VISA resource name"=w32) -> ("Error out"=→"Error out":errorcluster)  [unwired: 4 in]
    }
  }
